vi "纳清_校准量程设置.vi"(7 "探头":T1(ring), 8 "error in (no error)":errorcluster caption="错误输入（无错误）", 11 "校准量程":u16) -> (0 "error out":errorcluster caption="错误输出")   [LabVIEW 2022 SP3, in "斯坦道多参数.lvlib"]
uses:
  <vilib>/Plasmionique/MB Master/MB_Master/MB_Master.lvclass
  <vilib>/Plasmionique/MB Master/MB Master.lvlib
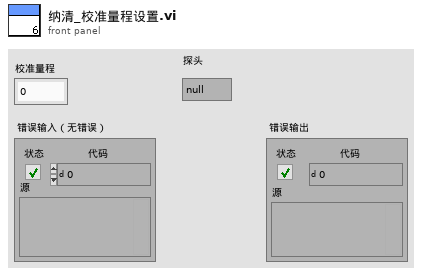
[diagram p1: front panel]
types:
  T1 = enum16{"null", "pH", "DO", "浊度", "电导率", "叶绿素a", "藻密度", "悬浮物"}
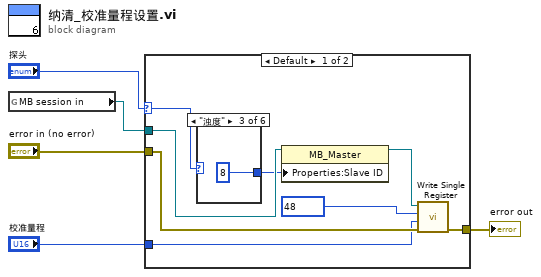
[diagram p0: block diagram]
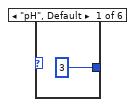
[diagram p2: hidden frame]
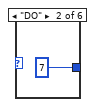
[diagram p3: hidden frame]
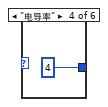
[diagram p4: hidden frame]
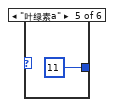
[diagram p5: hidden frame]
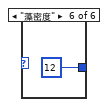
[diagram p6: hidden frame]
diagram:
  n1 = global read "多参数全局变量.vi" "MB session in"() -> (w2:refnum<class "MB_Master.lvclass">)
  n2 = case shown="Default" "探头" {
    selector: "探头" -> [w11 _]
    tunnel: "error in (no error)" -> [w10 w20]
    tunnel: [w7 w20] -> w4
    tunnel: w2 -> [w13 _]
    tunnel: "校准量程" -> [w6 _]
    frame Default {
      n3 = case shown="\"浊度\"" w11 {
        tunnel: [3 7 8 4 11 12] -> w12
        frame "pH", Default {
        }
        frame "DO" {
        }
        frame "浊度" {
        }
        frame "电导率" {
        }
        frame "叶绿素a" {
        }
        frame "藻密度" {
        }
      }
      n4 = property class="MB_Master"(reference=w13, "Properties:Slave ID"=w12) -> (reference out=w9:refnum<class "MB_Master.lvclass">)  [unwired: 1 in, 1 out]
      n5 = call <vilib>:"Write Single Register.vi"("error in (no error)"=w10, "value"=w6, "address"=u16 48 ("starting address"), "MB session in"=w9) -> ("error out"=w7:errorcluster)  [unwired: 6 in, 1 out]
    }
    frame "null" {
    }
  }
  "error out" <- w4
